vi "Hold feedback position for reinsertion..vi"(1 "Action(GET)":enum16{"GET", "SET"}(ring), 5 "Solenoid address inn":i16, 7 "Solenoid position in":dbl, 11 "error in (no error)":errorcluster) -> (6 "Solenoid address out":i16, 8 "Solenoid position out":dbl, 10 "Position updated":bool, 15 "error out":errorcluster)   [LabVIEW 2011]
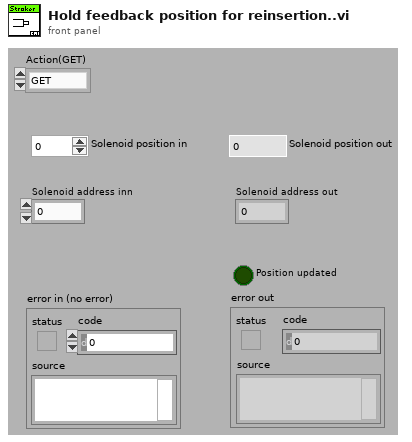
[diagram p1: front panel]
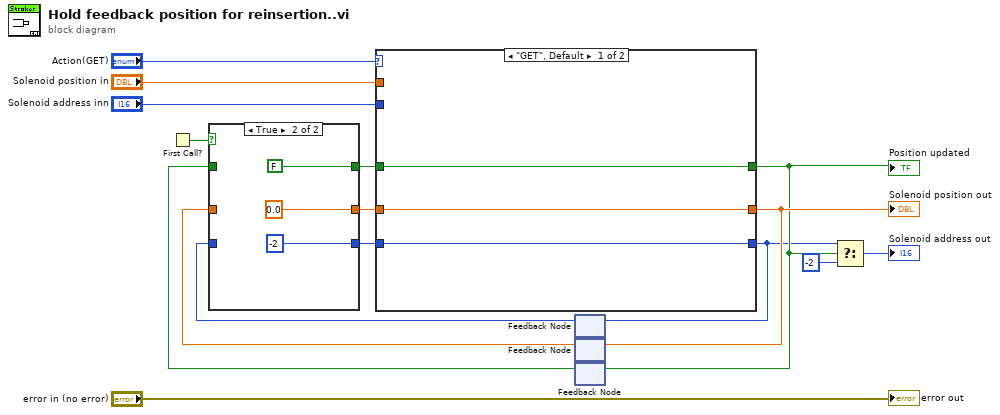
[diagram p0: block diagram]
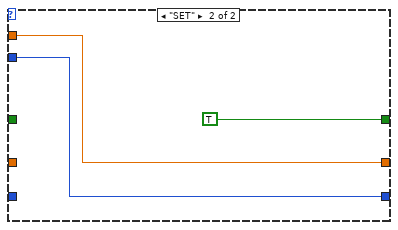
[diagram p3: hidden frame]
diagram:
  n1 = First Call?() -> (First Call?: T/F=w13:bool)
  n2 = feedback #1() -> (w6:i16)  [unwired: 1 in]
  n3 = feedback #2() -> (w14:dbl)  [unwired: 1 in]
  n4 = feedback #3() -> (w8:bool)  [unwired: 1 in]
  n5 = case shown="True" w13 {
    tunnel: w14 -> [w19 _]
    tunnel: [w19 0.0 ("Solenoid position")] -> w11
    tunnel: [w18 FALSE] -> w9
    tunnel: w8 -> [w18 _]
    tunnel: w6 -> [w17 _]
    tunnel: [w17 i16 -2 ("Solenoid address inn")] -> w5
    frame False {
    }
    frame True {
    }
  }
  n6 = case shown="\"GET\", Default" "Action(GET)" {
    tunnel: [w25 w28] -> w12
    tunnel: w11 -> [w25 _]
    tunnel: "Solenoid position in" -> [_ w28]
    tunnel: w9 -> [w24 _]
    tunnel: [w24 TRUE] -> w3
    tunnel: "Solenoid address inn" -> [_ w26]
    tunnel: [w23 w26] -> w2
    tunnel: w5 -> [w23 _]
    frame "GET", Default {
    }
    frame "SET" {
    }
  }
  "Solenoid position out" <- w12
  "Position updated" <- w3
  n7 = feedback-in #1(w2) -> ()
  n8 = feedback-in #2(w12) -> ()
  n9 = feedback-in #3(w3) -> ()
  n10 = Select(t=w2, s=w3, f=i16 -2) -> (s? t:f=→"Solenoid address out":i16)
  "error out" <- "error in (no error)"
